vi "Move XYZ.vi"(0 "PID Gains In":T1={"X PID"={"proportional gain (Kc)"=0.03, "integral time (Ti, min)"=0.0, "derivative time (Td, min)"=0.0}, "Y PID"={"proportional gain (Kc)"=0.03, "integral time (Ti, min)"=0.0, "derivative time (Td, min)"=0.0}, "Z PID"={"proportional gain (Kc)"=0.035, "integral time (Ti, min)"=0.0, "derivative time (Td, min)"=0.0}} {"Z PID"."derivative time (Td, min)" format="%.3f"; "Z PID"."integral time (Ti, min)" format="%.3f"; "Z PID"."proportional gain (Kc)" format="%.3f"; "Y PID"."derivative time (Td, min)" format="%.3f"; "Y PID"."integral time (Ti, min)" format="%.3f"; "Y PID"."proportional gain (Kc)" format="%.3f"; "X PID"."derivative time (Td, min)" format="%.3f"; "X PID"."integral time (Ti, min)" format="%.3f"; "X PID"."proportional gain (Kc)" format="%.3f"}, 5 "Y Target":dbl, 6 "X Target":dbl, 10 "Max Time":dbl=90.0, 11 "Gyro Target":dbl=-180.0, 12 "Movement":dbl=3.0, 14 "X Output Range":cluster{"output high":dbl, "output low":dbl}={"output high"=0.8, "output low"=-0.8}, 15 "X Stop Threshold":dbl=5.0, 16 "Y Output Range":cluster{"output high":dbl, "output low":dbl}={"output high"=0.8, "output low"=-0.8}, 17 "Y Stop Threshold":dbl=5.0, 18 "Z Output Range":cluster{"output high":dbl, "output low":dbl}={"output high"=0.8, "output low"=-0.8}, 19 "Z  Stop Threshold":dbl=8.0) -> ()   [LabVIEW 2018]
uses:
  Robot Global Data.vi
  SubSystems/Drive Train/Drive Train Global.vi
  SubSystems/Lift/Lift Global.vi
  SubSystems/Hatch Panel Intake/Hatch Panel Intake Global.vi
  <vilib>/addons/control/pid/pid.llb/PID (DBL).vi
  <vilib>/addons/control/pid/NI_PID_pid.lvlib
panel:
  in  "Minimum Time":u32=500
  in  "Settle Time":u32=2000
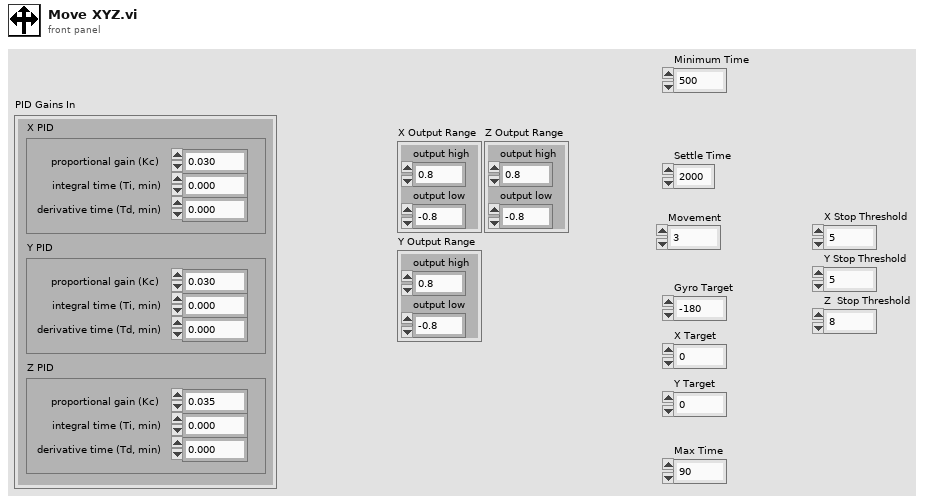
[diagram p1: front panel]
types:
  T1 = cluster{"X PID":cluster{"proportional gain (Kc)":dbl, "integral time (Ti, min)":dbl, "derivative time (Td, min)":dbl}, "Y PID":cluster{"proportional gain (Kc)":dbl, "integral time (Ti, min)":dbl, "derivative time (Td, min)":dbl}, "Z PID":cluster{"proportional gain (Kc)":dbl, "integral time (Ti, min)":dbl, "derivative time (Td, min)":dbl}}
  T2 = cluster{"proportional gain (Kc)":dbl, "integral time (Ti, min)":dbl, "derivative time (Td, min)":dbl}
  T3 = cluster{"Rollover":dbl, "Yaw":dbl, "Cont Yaw":dbl}
  T4 = cluster{"offsetAngle H":dbl, "offsetAngle V":dbl, "area":dbl, "skew":dbl, "validTarget":dbl, "latency":dbl}
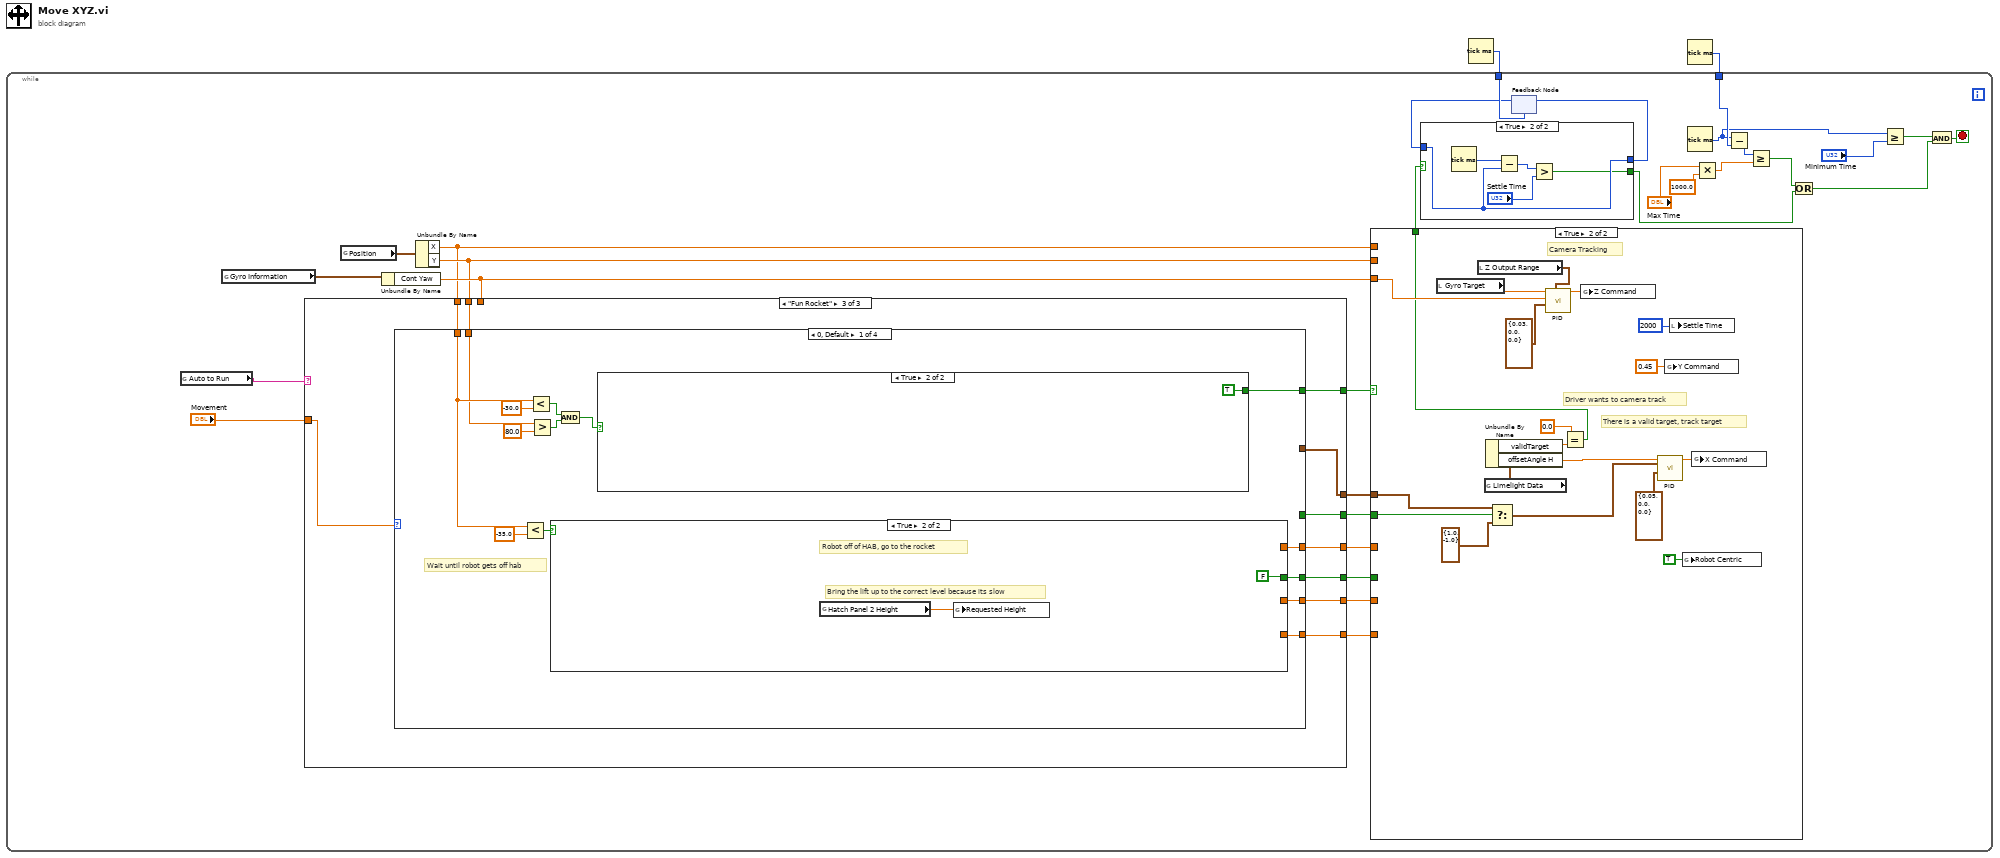
[diagram p0: block diagram]
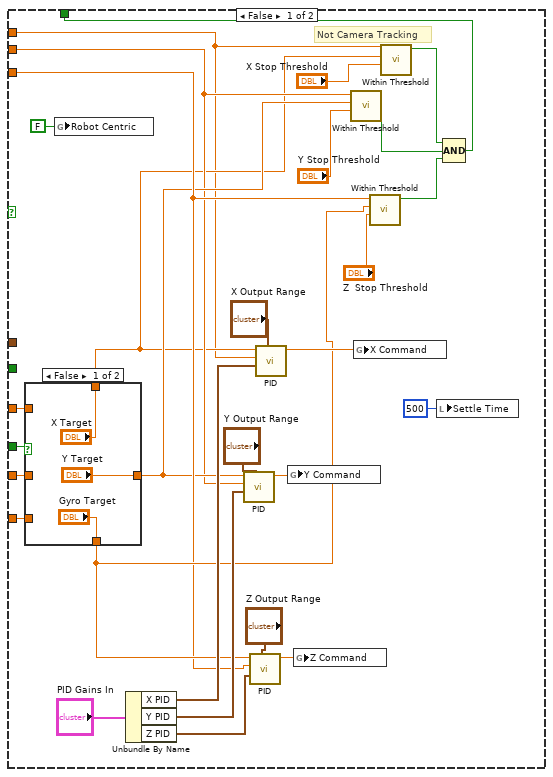
[diagram p2: hidden frame]
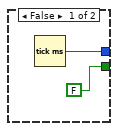
[diagram p4: hidden frame]
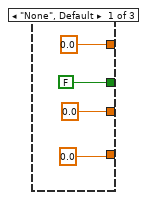
[diagram p5: hidden frame]
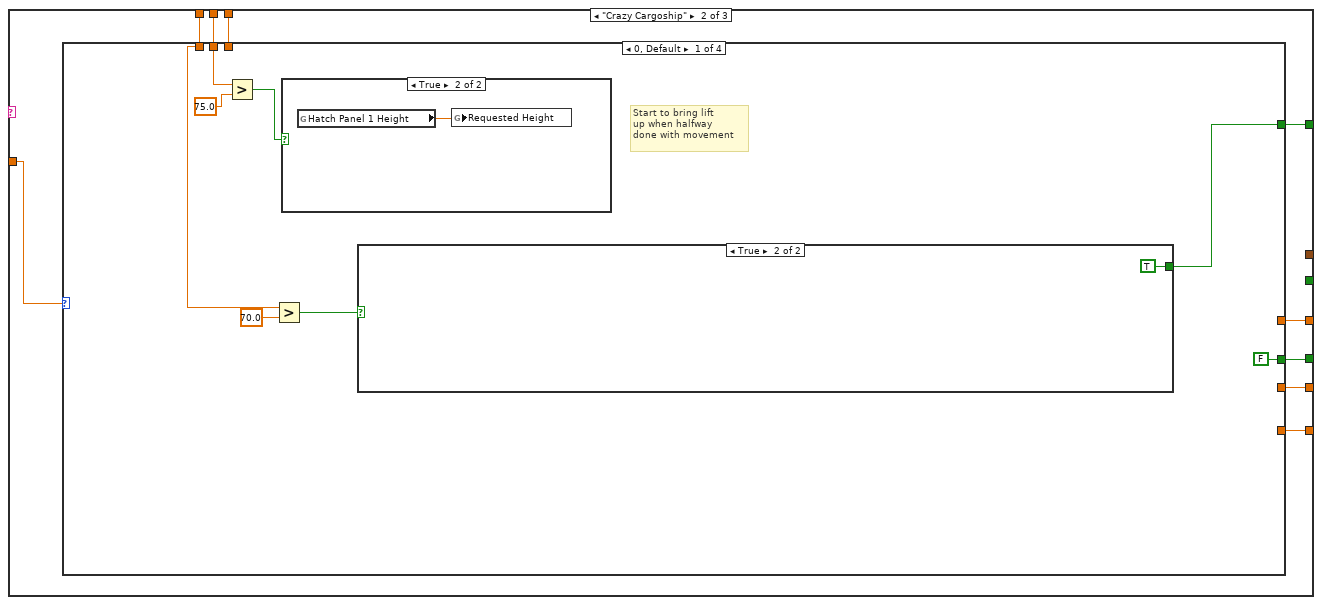
[diagram p6: hidden frame]
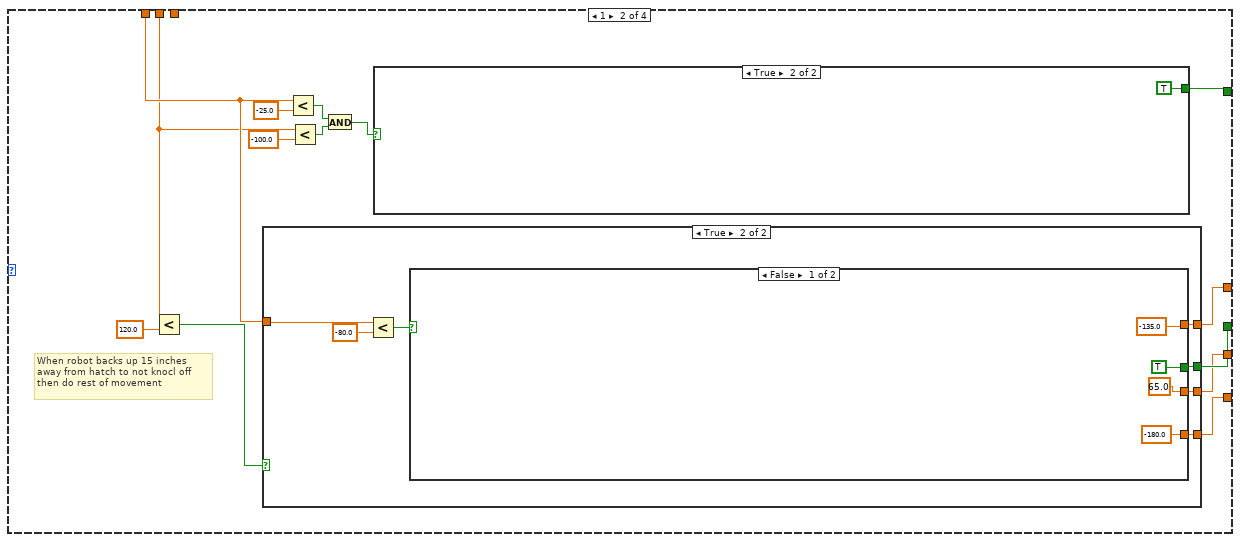
[diagram p9: hidden frame]
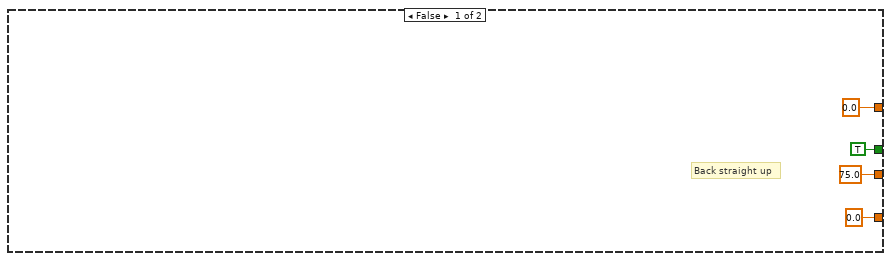
[diagram p11: hidden frame]
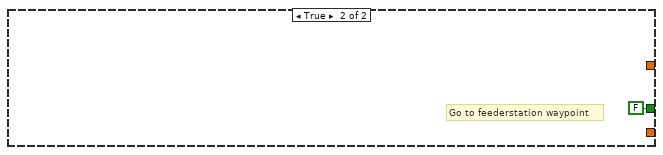
[diagram p12: hidden frame]
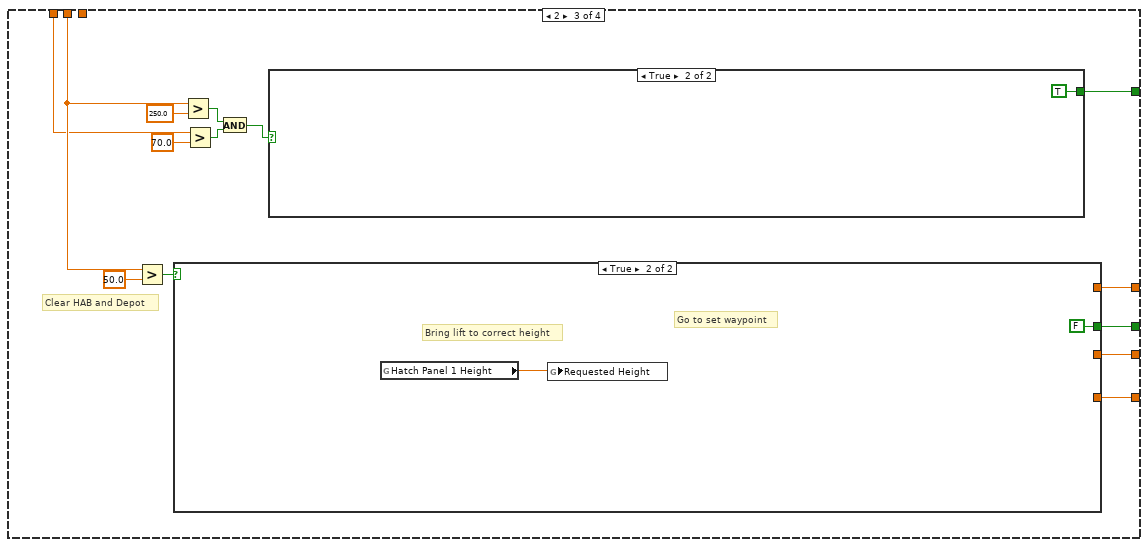
[diagram p13: hidden frame]
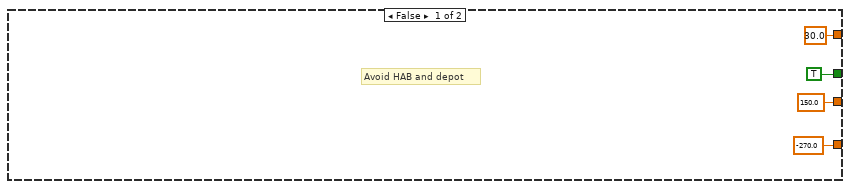
[diagram p15: hidden frame]
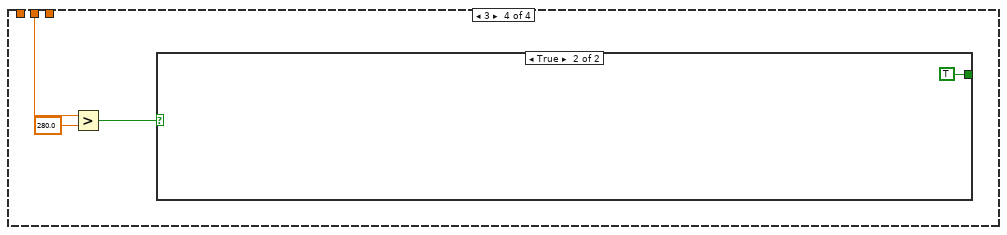
[diagram p16: hidden frame]
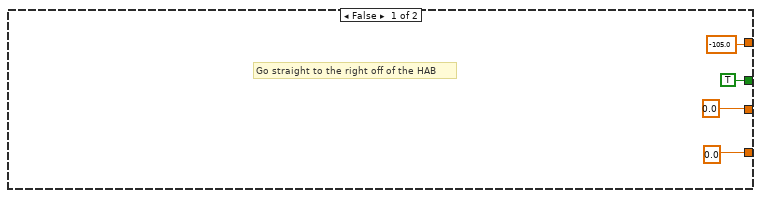
[diagram p19: hidden frame]
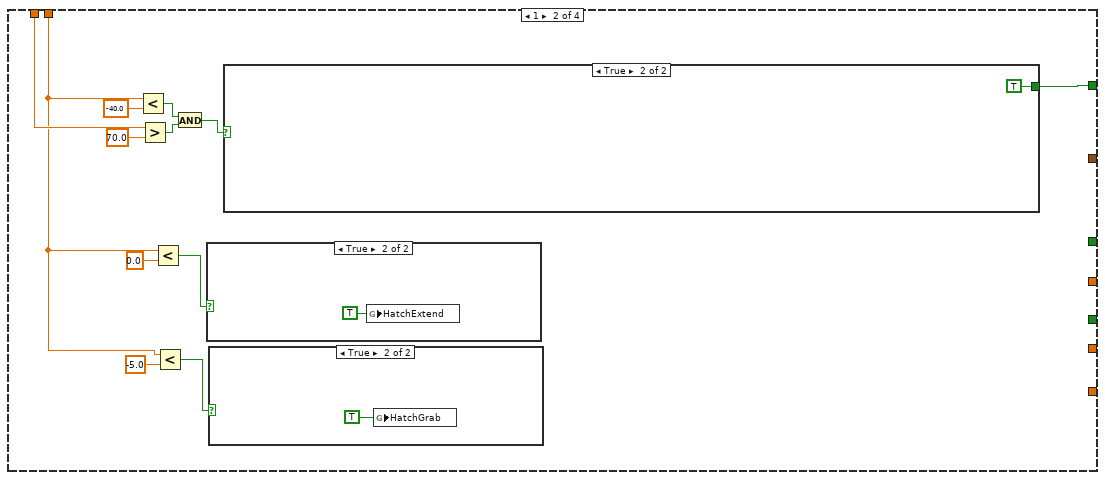
[diagram p20: hidden frame]
diagram:
  n1 = Tick Count (ms)() -> (millisecond timer value=w2:u32)
  n2 = Tick Count (ms)() -> (millisecond timer value=w1:u32)
  n3 = while {
    tunnel: w2 -> [w26]
    tunnel: w1 -> [w11]
    stop <- w10 stop-if-true
    n4 = global read "Robot Global Data.vi" "Auto to Run"() -> (w23:string)
    n5 = global read "Drive Train Global.vi" "Gyro Information"() -> (w20:T3)
    n6 = global read "Drive Train Global.vi" "Position"() -> (w22:cluster{"X":dbl, "Y":dbl})
    n7 = Unbundle By Name(w20) -> ("Cont Yaw"=w18:dbl)
    n8 = Unbundle By Name(w22) -> ("X"=w16:dbl, "Y"=w17:dbl)
    n9 = case shown="\"Fun Rocket\"" w23 {
      tunnel: [0.0 w101 w178] -> w32
      tunnel: [0.0 w100 w177] -> w31
      tunnel: [0.0 w99 w176] -> w30
      tunnel: w17 -> [_ w105 w181]
      tunnel: [FALSE w104 w179] -> w29
      tunnel: w16 -> [_ w102 w180]
      tunnel: "Movement" -> [_ w106 w182]
      tunnel: w18 -> [_ w103 _]
      tunnel: [_ w98 w175] -> w5
      tunnel: [_ _ w173] -> w4
      tunnel: [_ _ w174] -> w3
      frame "None", Default {
      }
      frame "Crazy Cargoship" {
        n10 = case shown="0, Default" w106 {
          tunnel: w105 -> [w114 w117 w149 w169]
          tunnel: [FALSE w128 w161 _] -> w104
          tunnel: w103 -> [_ _ _ _]
          tunnel: w102 -> [w107 w118 w148 _]
          tunnel: [_ w127 w158 _] -> w101
          tunnel: [_ w126 w157 _] -> w100
          tunnel: [_ w125 w156 _] -> w99
          tunnel: [w109 w119 w150 _] -> w98
          frame 0, Default {
            # "Start to bring lift\nup when halfway\ndone with movement"
            n11 = Greater?(x=w114, y=75.0) -> (0:w112:bool)
            n12 = Greater?(x=w107, y=70.0) -> (0:w108:bool)
            n13 = case shown="True" w112 {
              frame False {
              }
              frame True {
                n14 = global read "Lift Global.vi" "Hatch Panel 1 Height"() -> (w116:dbl)
                n15 = global write "Lift Global.vi" "Requested Height"(w116) -> ()
              }
            }
            n16 = case shown="True" w108 {
              tunnel: [_ TRUE] -> w109
              frame False {
              }
              frame True {
              }
            }
          }
          frame 1 {
            # "When robot backs up 15 inches\naway from hatch to not knocl off\nthen do rest of movement"
            n17 = Less?(x=w117, y=120.0) -> (x < y?=w130:bool)
            n18 = case shown="True" w130 {
              tunnel: [TRUE w142] -> w128
              tunnel: [0.0 w138] -> w127
              tunnel: [75.0 w137] -> w126
              tunnel: [0.0 w136] -> w125
              tunnel: w118 -> [_ w139]
              frame False {
                # "Back straight up"
              }
              frame True {
                n19 = Less?(x=w139, y=-80.0) -> (x < y?=w140:bool)
                n20 = case shown="False" w140 {
                  tunnel: [TRUE FALSE] -> w142
                  tunnel: [-135.0 _] -> w138
                  tunnel: [65.0 _] -> w137
                  tunnel: [-180.0 _] -> w136
                  frame False {
                  }
                  frame True {
                    # "Go to feederstation waypoint"
                  }
                }
              }
            }
            n21 = Less?(x=w118, y=-25.0) -> (x < y?=w122:bool)
            n22 = Less?(x=w117, y=-100.0) -> (x < y?=w121:bool)
            n23 = And(x=w122, y=w121) -> (x .and. y?=w120:bool)
            n24 = case shown="True" w120 {
              tunnel: [_ TRUE] -> w119
              frame False {
              }
              frame True {
              }
            }
          }
          frame 2 {
            # "Clear HAB and Depot"
            n25 = Greater?(x=w149, y=50.0) -> (0:w160:bool)
            n26 = case shown="True" w160 {
              tunnel: [TRUE FALSE] -> w161
              tunnel: [30.0 _] -> w158
              tunnel: [150.0 _] -> w157
              tunnel: [-270.0 _] -> w156
              frame False {
                # "Avoid HAB and depot"
              }
              frame True {
                # "Bring lift to correct height"
                # "Go to set waypoint"
                n27 = global read "Lift Global.vi" "Hatch Panel 1 Height"() -> (w167:dbl)
                n28 = global write "Lift Global.vi" "Requested Height"(w167) -> ()
              }
            }
            n29 = Greater?(x=w149, y=250.0) -> (0:w153:bool)
            n30 = Greater?(x=w148, y=70.0) -> (0:w152:bool)
            n31 = And(x=w153, y=w152) -> (x .and. y?=w151:bool)
            n32 = case shown="True" w151 {
              tunnel: [_ TRUE] -> w150
              frame False {
              }
              frame True {
              }
            }
          }
          frame 3 {
            n33 = Greater?(x=w169, y=280.0) -> (0:w170:bool)
            n34 = case shown="True" w170 {
              tunnel: [_ TRUE] -> _
              frame False {
              }
              frame True {
              }
            }
          }
        }
      }
      frame "Fun Rocket" {
        n35 = case shown="0, Default" w182 {
          tunnel: w181 -> [w189 w204 w221 w228]
          tunnel: w180 -> [w190 w209 _ _]
          tunnel: [w194 _ _ _] -> w179
          tunnel: [w193 _ _ _] -> w178
          tunnel: [w192 _ _ _] -> w177
          tunnel: [w191 _ _ _] -> w176
          tunnel: [w183 w210 w223 w230] -> w175
          tunnel: [_ _ w220 _] -> w174
          tunnel: [_ _ w219 _] -> w173
          frame 0, Default {
            # "Wait until robot gets off hab"
            n36 = Less?(x=w190, y=-35.0) -> (x < y?=w196:bool)
            n37 = Less?(x=w190, y=-30.0) -> (x < y?=w186:bool)
            n38 = Greater?(x=w189, y=80.0) -> (0:w185:bool)
            n39 = case shown="True" w196 {
              tunnel: [TRUE FALSE] -> w194
              tunnel: [-105.0 _] -> w193
              tunnel: [0.0 _] -> w192
              tunnel: [0.0 _] -> w191
              frame False {
                # "Go straight to the right off of the HAB"
              }
              frame True {
                # "Bring the lift up to the correct level because its slow"
                # "Robot off of HAB, go to the rocket"
                n40 = global read "Lift Global.vi" "Hatch Panel 2 Height"() -> (w202:dbl)
                n41 = global write "Lift Global.vi" "Requested Height"(w202) -> ()
              }
            }
            n42 = And(x=w186, y=w185) -> (x .and. y?=w184:bool)
            n43 = case shown="True" w184 {
              tunnel: [_ TRUE] -> w183
              frame False {
              }
              frame True {
              }
            }
          }
          frame 1 {
            n44 = Less?(x=w204, y=-40.0) -> (x < y?=w213:bool)
            n45 = Greater?(x=w209, y=70.0) -> (0:w212:bool)
            n46 = Less?(x=w204, y=0.0) -> (x < y?=w207:bool)
            n47 = Less?(x=w204, y=-5.0) -> (x < y?=w206:bool)
            n48 = And(x=w213, y=w212) -> (x .and. y?=w211:bool)
            n49 = case shown="True" w207 {
              frame False {
              }
              frame True {
                n50 = global write "Hatch Panel Intake Global.vi" "HatchExtend"(TRUE ("HatchExtend")) -> ()
              }
            }
            n51 = case shown="True" w206 {
              frame False {
              }
              frame True {
                n52 = global write "Hatch Panel Intake Global.vi" "HatchGrab"(TRUE ("HatchExtend")) -> ()
              }
            }
            n53 = case shown="True" w211 {
              tunnel: [_ TRUE] -> w210
              frame False {
              }
              frame True {
              }
            }
          }
          frame 2 {
            # "NEEDS TO BACK UP THEN TURN"
            n54 = Greater?(x=w221, y=150.0) -> (0:w222:bool)
            n55 = case shown="True" w222 {
              tunnel: [_ TRUE] -> w223
              tunnel: [_ TRUE] -> w220
              tunnel: [_ cluster{"output high":dbl, "output low":dbl} {"output high"=0.7, "output low"=-0.7} ("output range")] -> w219
              frame False {
              }
              frame True {
              }
            }
          }
          frame 3 {
            n56 = Less?(x=w228, y=30.0) -> (x < y?=w229:bool)
            n57 = case shown="True" w229 {
              tunnel: [_ TRUE] -> w230
              frame False {
              }
              frame True {
              }
            }
          }
        }
      }
    }
    n58 = case shown="True" w5 {
      tunnel: w32 -> [w54 _]
      tunnel: w31 -> [w53 _]
      tunnel: w30 -> [w52 _]
      tunnel: w29 -> [w51 _]
      tunnel: [w35 w73] -> w19
      tunnel: w18 -> [w45 w77]
      tunnel: w17 -> [w41 _]
      tunnel: w16 -> [w37 _]
      tunnel: w4 -> [_ w70]
      tunnel: w3 -> [_ w69]
      frame False {
        # "Not Camera Tracking"
        n59 = case shown="False" w51 {
          tunnel: ["X Target" w67] -> w38
          tunnel: ["Y Target" w66] -> w42
          tunnel: ["Gyro Target" w65] -> w46
          tunnel: w54 -> [_ w67]
          tunnel: w53 -> [_ w66]
          tunnel: w52 -> [_ w65]
          frame False {
          }
          frame True {
          }
        }
        n60 = global write "Drive Train Global.vi" "Robot Centric"(FALSE ("Robot Centric")) -> ()
        n61 = Unbundle By Name("PID Gains In") -> ("X PID"=w59:T2, "Y PID"=w58:T2, "Z PID"=w57:T2)
        n62 = call-poly <vilib>:"PID.vi"("output range"="Y Output Range", "PID gains"=w58, "process variable"=w41, "setpoint"=w42) -> ("output"=w48:dbl)  [unwired: 6 in, 1 out]
        n63 = call-poly <vilib>:"PID.vi"("output range"="Z Output Range", "PID gains"=w57, "process variable"=w45, "setpoint"=w46) -> ("output"=w49:dbl)  [unwired: 6 in, 1 out]
        n64 = call-poly <vilib>:"PID.vi"("output range"="X Output Range", "PID gains"=w59, "process variable"=w37, "setpoint"=w38) -> ("output"=w50:dbl)  [unwired: 6 in, 1 out]
        n65 = global write "Drive Train Global.vi" "Y Command"(w48) -> ()
        n66 = global write "Drive Train Global.vi" "Z Command"(w49) -> ()
        n67 = call "Within Threshold.vi"("Threshold"="Y Stop Threshold", "Center"=w42, "Value"=w41) -> ("Within Threshold?"=w43:bool)  [unwired: 8 in]
        n68 = global write "Drive Train Global.vi" "X Command"(w50) -> ()
        n69 = call "Within Threshold.vi"("Threshold"="Z  Stop Threshold", "Center"=w46, "Value"=w45) -> ("Within Threshold?"=w47:bool)  [unwired: 8 in]
        n70 = call "Within Threshold.vi"("Threshold"="X Stop Threshold", "Center"=w38, "Value"=w37) -> ("Within Threshold?"=w39:bool)  [unwired: 8 in]
        n71 = local write "Settle Time"(u32 500 ("Settle Time")) -> ()
        n72 = Compound Arithmetic op=AND(w39, w43, w47) -> (w35:bool)
      }
      frame True {
        # "There is a valid target, track target"
        # "Driver wants to camera track"
        # "Camera Tracking"
        n73 = local read "Gyro Target"() -> (w78:dbl)
        n74 = local read "Z Output Range"() -> (w79:cluster{"output high":dbl, "output low":dbl})
        n75 = global read "Robot Global Data.vi" "Limelight Data"() -> (w84:T4)
        n76 = Unbundle By Name(w84) -> ("validTarget"=w75:dbl, "offsetAngle H"=w83:dbl)
        n77 = Select(t=w70, s=w69, f=cluster{"output high":dbl, "output low":dbl} {"output high"=1.0, "output low"=-1.0} ("output range")) -> (s? t:f=w71:cluster{"output high":dbl, "output low":dbl})
        n78 = call-poly <vilib>:"PID.vi"("output range"=w79, "PID gains"=T2 {"proportional gain (Kc)"=0.03, "integral time (Ti, min)"=0.0, "derivative time (Td, min)"=0.0}, "process variable"=w77, "setpoint"=w78) -> ("output"=w80:dbl)  [unwired: 6 in, 1 out]
        n79 = Equal?(x=0.0, y=w75) -> (x = y?=w73:bool)
        n80 = global write "Drive Train Global.vi" "Z Command"(w80) -> ()
        n81 = call-poly <vilib>:"PID.vi"("output range"=w71, "PID gains"=T2 {"proportional gain (Kc)"=0.05, "integral time (Ti, min)"=0.0, "derivative time (Td, min)"=0.0} ("Camera Tracking"), "setpoint"=w83) -> ("output"=w85:dbl)  [unwired: 7 in, 1 out]
        n82 = global write "Drive Train Global.vi" "Y Command"(0.45 ("Y Command")) -> ()
        n83 = local write "Settle Time"(u32 2000 ("Settle Time")) -> ()
        n84 = global write "Drive Train Global.vi" "Robot Centric"(TRUE ("Robot Centric")) -> ()
        n85 = global write "Drive Train Global.vi" "X Command"(w85) -> ()
      }
    }
    n86 = feedback #1(w26) -> (w25:u32)
    n87 = case shown="True" w19 {
      tunnel: [w88 w91] -> w27
      tunnel: w25 -> [_ w91]
      tunnel: [FALSE w90] -> w24
      frame False {
        n88 = Tick Count (ms)() -> (millisecond timer value=w88:u32)
      }
      frame True {
        n89 = Tick Count (ms)() -> (millisecond timer value=w93:u32)
        n90 = Subtract(x=w93, y=w91) -> (x-y=w92:u32)
        n91 = Greater?(x=w92, y="Settle Time") -> (0:w90:bool)
      }
    }
    n92 = feedback-in #1(w27) -> ()
    n93 = Tick Count (ms)() -> (millisecond timer value=w9:u32)
    n94 = Multiply(x="Max Time", y=1000.0) -> (x*y=w14:dbl)
    n95 = Subtract(x=w9, y=w11) -> (x-y=w15:u32)
    n96 = Greater Or Equal?(x=w15, y=w14) -> (x >= y?=w28:bool)
    n97 = Or(x=w28, y=w24) -> (x .or. y?=w6:bool)
    n98 = Greater Or Equal?(x=w9, y="Minimum Time") -> (x >= y?=w7:bool)
    n99 = And(x=w7, y=w6) -> (x .and. y?=w10:bool)
  }
